vi "RSZVB Configure Calibration Standard With Label.vi"(5 "Approximation (Open)":i32(ring) items=["Open", "Short", "Match"], 6 "Polynomial Coefficients":T2 {"Residual Inductances" format="%^.3e"; "Capacitances" format="%^.3e"}, 7 "Settings":T1 {"Z0" format="%^.3e"; "Loss" format="%^.3e"; "Electrical Length" format="%^.3e"; "Max. Freq [Hz]" format="%^.3e"; "Min. Freq [Hz]" format="%^.3e"}, 8 "error in (no error)":errorcluster {"code" format="%.0x"}, 9 "Identifiers":T3, 10 "Standard (Through (MM))":i32(ring) items=["Through (MM)", "Through (FF)", "Through (MF)", "Line 1 (MM)", "Line 1 (FF)", "Line 1 (MF)", "Offset short (sexless)", "Offset short 1 (M)", "Offset short 1 (F)", "Attenuation (MM)", "Attenuation (FF)", "Attenuation (MF)", "Symm Network (MM)", "Symm Network (FF)", "Symm Network (MF)", "Open (M)", "Open (F)", "Short (M)", "Short (F)", "Reflect (M)", "Reflect (F)", "Match (M)", "Match (F)", "Sliding Match (M)", "Sliding Match (F)", "Line 2 (MM)", "Line 2 (FF)", "Line 2 (MF)", "Line 3 (MM)", "Line 3 (FF)", "Line 3 (MF)", "Offset short 2 (M)", "Offset short 2 (F)", "Offset short 3 (M)", "Offset short 3 (F)"], 11 "VISA session":refnum<visa-resource-name>) -> (0 "error out":errorcluster {"code" format="%.0x"}, 3 "dup VISA session":refnum<visa-resource-name>)   [LabVIEW 2011]
doc: "This VI defines the parameters of a non-ideal 1 port or 2-port calibration standard <std_type>\n\nAttribute(s):\n-\n\nRemote-control command(s):\n[SENSe<Ch>:]CORRection:CKIT:<std_type>:WLABel"
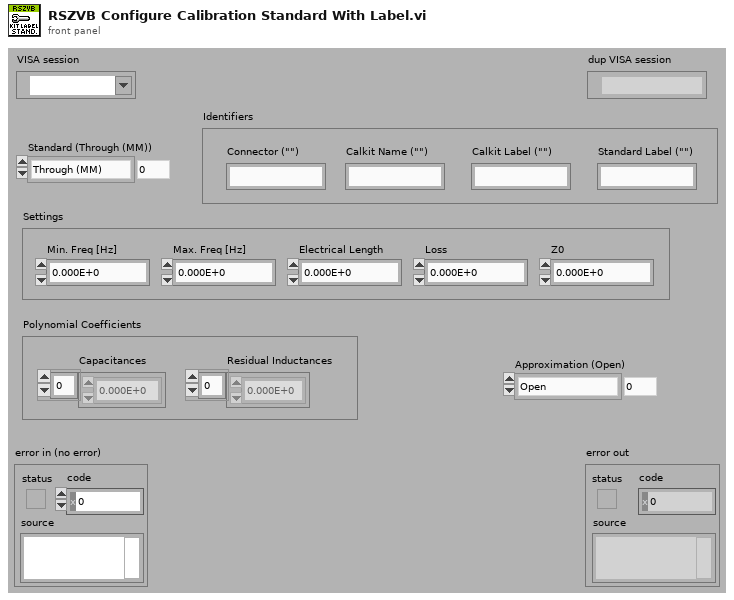
[diagram p1: front panel]
types:
  T1 = cluster{"Min. Freq [Hz]":dbl, "Max. Freq [Hz]":dbl, "Electrical Length":dbl, "Loss":dbl, "Z0":dbl}
  T2 = cluster{"Capacitances":dbl[], "Residual Inductances":dbl[]}
  T3 = cluster{"Connector (\"\")":string, "Calkit Name (\"\")":string, "Calkit Label (\"\")":string, "Standard Label (\"\")":string}
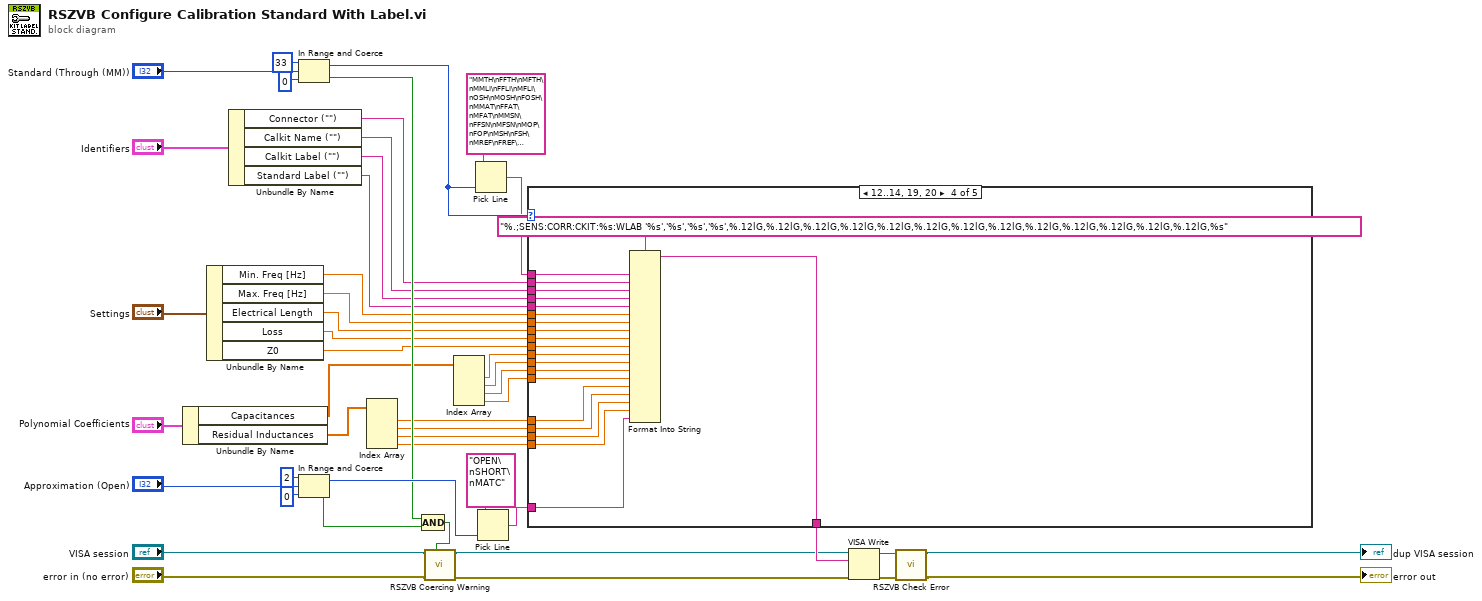
[diagram p0: block diagram]
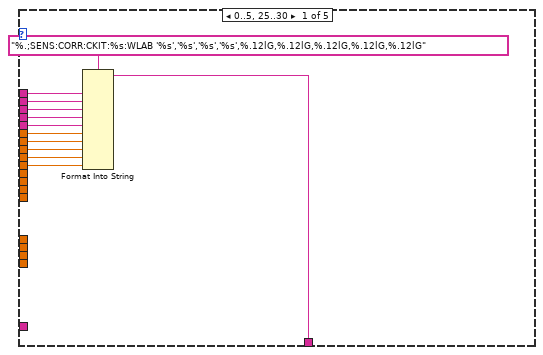
[diagram p2: hidden frame]
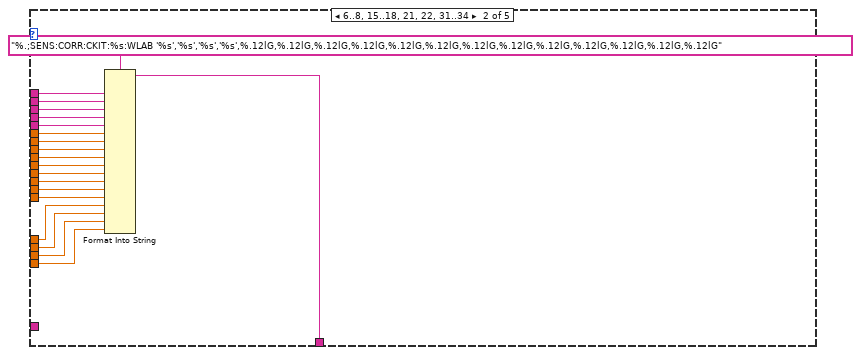
[diagram p3: hidden frame]
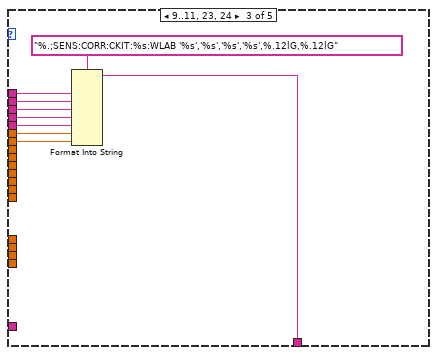
[diagram p4: hidden frame]
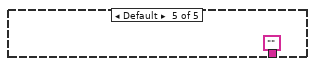
[diagram p5: hidden frame]
diagram:
  n1 = Unbundle By Name("Polynomial Coefficients") -> ("Capacitances"=w25:dbl[], "Residual Inductances"=w20:dbl[])
  n2 = Unbundle By Name("Settings") -> ("Min. Freq [Hz]"=w30:dbl, "Max. Freq [Hz]"=w29:dbl, "Electrical Length"=w28:dbl, "Loss"=w27:dbl, "Z0"=w26:dbl)
  n3 = Unbundle By Name("Identifiers") -> ("Connector (\"\")"=w31:string, "Calkit Name (\"\")"=w32:string, "Calkit Label (\"\")"=w33:string, "Standard Label (\"\")"=w34:string)
  n4 = In Range and Coerce(upper limit=33 ("lower limit"), x="Standard (Through (MM))", lower limit=0) -> (coerced(x)=w40:i32, In Range?=w36:bool)
  n5 = In Range and Coerce(upper limit=2 ("lower limit"), x="Approximation (Open)", lower limit=0) -> (coerced(x)=w39:i32, In Range?=w35:bool)
  n6 = Index Array(array=w20) -> (element #1=w16:dbl, element #2=w17:dbl, element #3=w18:dbl, element #4=w19:dbl)  [unwired: 4 in]
  n7 = Compound Arithmetic op=AND(w36, w35) -> (w2:bool)
  n8 = call "RSZVB Coercing Warning.vi"("In Range?"=w2, "error in (no error)"="error in (no error)", "VISA session"="VISA session") -> ("error out"=w15:errorcluster, "dup VISA session"=w12:refnum<visa-resource-name>)  [unwired: 7 in]
  n9 = Index Array(array=w25) -> (element #1=w24:dbl, element #2=w23:dbl, element #3=w22:dbl, element #4=w21:dbl)  [unwired: 4 in]
  n10 = Pick Line(multi-line string="MMTH\nFFTH\nMFTH\nMMLI\nFFLI\nMFLI\nOSH\nMOSH\nFOSH\nMMAT\nFFAT\nMFAT\nMMSN\nFFSN\nMFSN\nMOP\nFOP\nMSH\nFSH\nMREF\nFREF\nMMTC\nFMTC\nMSM\nFSM\nMMLI2\nFFLI2\nMFLI2\nMMLI3\nFFLI3\nMFLI3\nMOSHORT2\nFOSHORT2\nMOSHORT3\nFOSHORT3", line index=w40) -> (output string=w37:string)  [unwired: 1 in]
  n11 = Pick Line(multi-line string="OPEN\nSHORT\nMATC", line index=w39) -> (output string=w42:string)  [unwired: 1 in]
  n12 = case shown="12..14, 19, 20" w40 {
    tunnel: w42 -> [_ _ _ w98 _]
    tunnel: [w56 w77 w86 w107 ""] -> w38
    tunnel: w37 -> [w55 w72 w85 w106 _]
    tunnel: w31 -> [w58 w73 w84 w105 _]
    tunnel: w33 -> [w53 w75 w82 w103 _]
    tunnel: w34 -> [w52 w76 w81 w102 _]
    tunnel: w30 -> [w51 w71 w80 w101 _]
    tunnel: w29 -> [w50 w70 w79 w100 _]
    tunnel: w28 -> [w49 w69 _ w99 _]
    tunnel: w27 -> [w48 w68 _ w88 _]
    tunnel: w32 -> [w54 w74 w83 w104 _]
    tunnel: w26 -> [w47 w67 _ w89 _]
    tunnel: w24 -> [_ w66 _ w90 _]
    tunnel: w23 -> [_ w65 _ w91 _]
    tunnel: w22 -> [_ w64 _ w92 _]
    tunnel: w21 -> [_ w63 _ w93 _]
    tunnel: w19 -> [_ w59 _ w97 _]
    tunnel: w18 -> [_ w60 _ w96 _]
    tunnel: w17 -> [_ w61 _ w95 _]
    tunnel: w16 -> [_ w62 _ w94 _]
    frame 0..5, 25..30 {
      n13 = Format Into String(format string="%.;SENS:CORR:CKIT:%s:WLAB '%s','%s','%s','%s',%.12lG,%.12lG,%.12lG,%.12lG,%.12lG", w55, w58, w54, w53, w52, w51, w50, w49, w48, w47) -> (resulting string=w56:string)  [unwired: 2 in, 1 out]
    }
    frame 6..8, 15..18, 21, 22, 31..34 {
      n14 = Format Into String(format string="%.;SENS:CORR:CKIT:%s:WLAB '%s','%s','%s','%s',%.12lG,%.12lG,%.12lG,%.12lG,%.12lG,%.12lG,%.12lG,%.12lG,%.12lG,%.12lG,%.12lG,%.12lG,%.12lG", w72, w73, w74, w75, w76, w71, w70, w69, w68, w67, w66, w65, w64, w63, w62, w61, w60, w59) -> (resulting string=w77:string)  [unwired: 2 in, 1 out]
    }
    frame 9..11, 23, 24 {
      n15 = Format Into String(format string="%.;SENS:CORR:CKIT:%s:WLAB '%s','%s','%s','%s',%.12lG,%.12lG", w85, w84, w83, w82, w81, w80, w79) -> (resulting string=w86:string)  [unwired: 2 in, 1 out]
    }
    frame 12..14, 19, 20 {
      n16 = Format Into String(format string="%.;SENS:CORR:CKIT:%s:WLAB '%s','%s','%s','%s',%.12lG,%.12lG,%.12lG,%.12lG,%.12lG,%.12lG,%.12lG,%.12lG,%.12lG,%.12lG,%.12lG,%.12lG,%.12lG,%s", w106, w105, w104, w103, w102, w101, w100, w99, w88, w89, w90, w91, w92, w93, w94, w95, w96, w97, w98) -> (resulting string=w107:string)  [unwired: 2 in, 1 out]
    }
    frame Default {
      (unwired) ""
    }
  }
  n17 = VISA Write(VISA resource name=w12, write buffer=w38, error in (no error)=w15) -> (VISA resource name out=w8:refnum<visa-resource-name>, error out=w9:errorcluster)  [unwired: 1 out]
  n18 = call "RSZVB Check Error.vi"("error in (no error)"=w9, "VISA session"=w8) -> ("error out"=→"error out":errorcluster, "dup VISA session"=→"dup VISA session":refnum<visa-resource-name>)  [unwired: 8 in]
